vi "Gyro Global.vi"() -> ()   [LabVIEW 2015]
panel:
  in  "Gyro 2 Data":cluster{"Rate":dbl, "Angle":dbl, "Gain":dbl}={"Rate"=0.0, "Angle"=0.0, "Gain"=0.07}
  in  "Gyro 1 Data":cluster{"Rate":dbl, "Angle":dbl, "Gain":dbl}={"Rate"=0.0, "Angle"=0.0, "Gain"=0.07}
  out "VisitedEnabled":bool
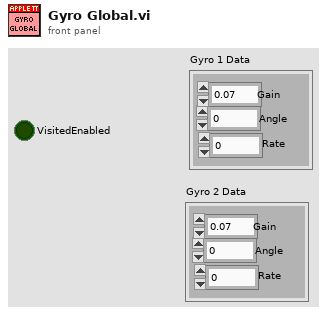
[diagram p1: front panel]
diagram:
